vi "Script Control To ConPane.vi"(4 "Pane":refnum<vi>, 6 "VI Ref":refnum<vi>, 7 "Terminal Index":i32, 8 "error in":errorcluster, 9 "Wire Rule":T1(ring), 10 "Control":refnum<vi>) -> (0 "error out":errorcluster, 2 "Control":refnum<vi>)   [LabVIEW 2025, in "_Rescript.lvlib" / "_Rescript.lvclass"]
uses:
  _Rescript.lvclass
  <vilib>/Utility/miscctls.llb/LVPositionTypeDef.ctl
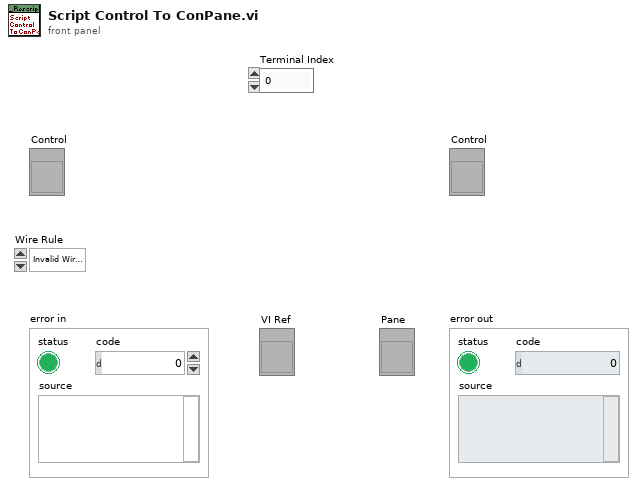
[diagram p1: front panel]
types:
  T1 = enum16{"Invalid Wire Rule", "Required", "Recommended", "Optional", "Dynamic Dispatch"}
  T2 = typedef "LVPositionTypeDef.ctl" = cluster{"Left":i32, "Top":i32}
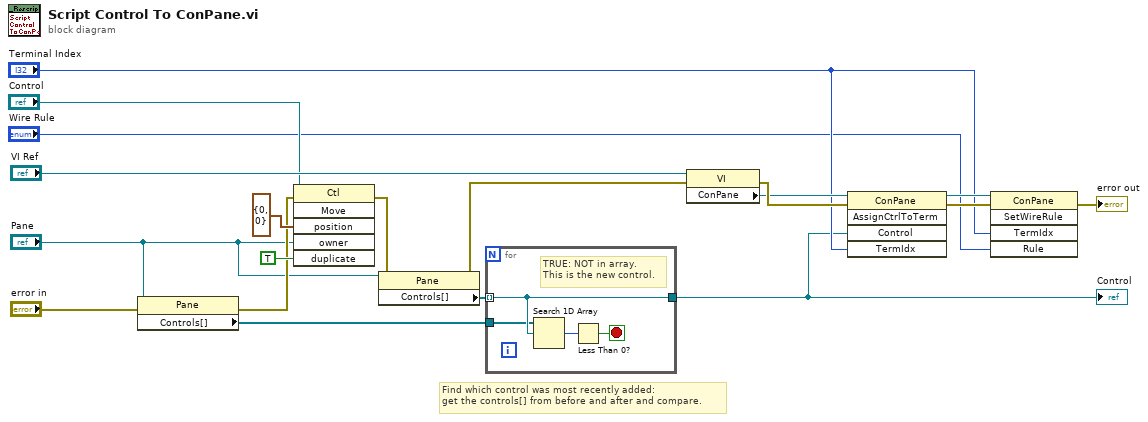
[diagram p0: block diagram]
diagram:
  # "Find which control was most recently added:\nget the controls[] from before and after and compare."
  n1 = property class="Pane"(reference="Pane", error in="error in") -> (error out=w13:errorcluster, "Controls[]"=w11:refnum<vi>[])  [unwired: 1 out]
  n2 = invoke class="Ctl" method="Move"(reference="Control", error in=w13, "position"=T2 {"Left"=0, "Top"=0}, "owner"="Pane", "duplicate"=TRUE ("Duplicate? (F)")) -> (error out=w10:errorcluster)  [unwired: 1 in, 5 out]
  n3 = property class="Pane"(reference="Pane", error in=w10) -> (error out=w9:errorcluster, "Controls[]"=w12:refnum<vi>[])  [unwired: 1 out]
  n4 = for {
    tunnel: w12 -> [w23] mode=indexing
    tunnel: w11 -> [w22]
    tunnel: [w23] -> w3
    stop <- w20 stop-if-true
    # "TRUE: NOT in array.\nThis is the new control."
    n5 = Search 1D Array(1D array=w22, element=w23) -> (index of element=w21:i32)  [unwired: 1 in]
    n6 = Less Than 0?(x=w21) -> (x < 0?=w20:bool)
  }
  "Control" <- w3
  n7 = property class="VI"(reference="VI Ref", error in=w9) -> (error out=w16:errorcluster, "ConPane"=w14:refnum<vi>)  [unwired: 1 out]
  n8 = invoke class="ConPane" method="AssignCtrlToTerm"(reference=w14, error in=w16, "Control"=w3, "TermIdx"="Terminal Index") -> (reference out=w17:refnum<vi>, error out=w15:errorcluster)  [unwired: 1 in, 3 out]
  n9 = invoke class="ConPane" method="SetWireRule"(reference=w17, error in=w15, "TermIdx"="Terminal Index", "Rule"="Wire Rule") -> (error out=→"error out":errorcluster)  [unwired: 1 in, 4 out]
